vi "电源FGV.vi"(8 "error in (no error)":errorcluster caption="错误输入（无错误）", 9 "Voltage":dbl=2.7, 10 "枚举":T1) -> (0 "error out":errorcluster caption="错误输出", 3 "VISA资源名称输出":refnum<visa-resource-name>)   [LabVIEW 2012]
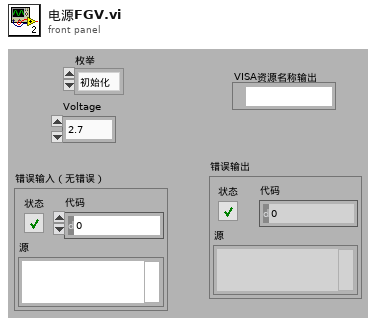
[diagram p1: front panel]
types:
  T1 = typedef "控件 3.ctl" = enum16{"初始化", "读取", "写入", "退出"}
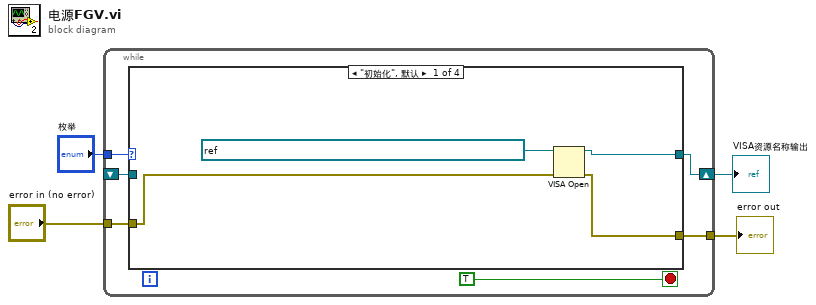
[diagram p0: block diagram]
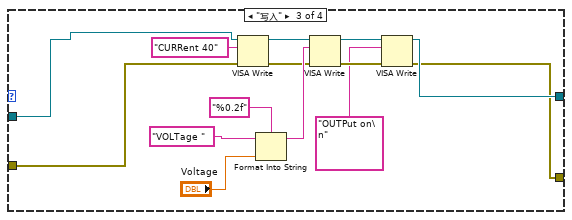
[diagram p3: hidden frame]
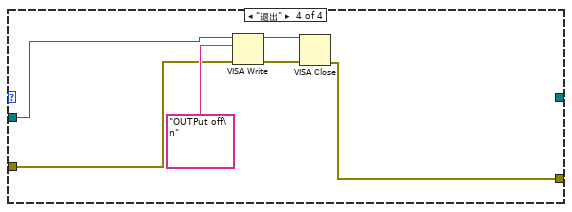
[diagram p4: hidden frame]
diagram:
  n1 = while {
    tunnel: "枚举" -> [w9]
    shift-right: [w8] -> w3
    shift-left: _ -> [w7]
    tunnel: "error in (no error)" -> [w6]
    tunnel: [w5] -> w1
    stop <- TRUE stop-if-true
    n2 = case shown="\"初始化\", 默认" w9 {
      tunnel: [w13 w16 w23 _] -> w8
      tunnel: w7 -> [_ w16 w18 w33]
      tunnel: w6 -> [w12 w15 w17 w32]
      tunnel: [w11 w15 w22 w31] -> w5
      frame "初始化", Default {
        n3 = VISA Open(error in (no error)=w12, VISA resource name=refnum<visa-resource-name> "USB0::0xFFFF::0x6500::600264012697220016::INSTR" ("VISA资源名称")) -> (VISA resource name=w13:refnum<visa-resource-name>, error out=w11:errorcluster)  [unwired: 3 in]
      }
      frame "读取" {
      }
      frame "写入" {
        n4 = VISA Write(VISA resource name=w18, write buffer="CURRent 40" ("写入缓冲区"), error in (no error)=w17) -> (VISA resource name out=w20:refnum<visa-resource-name>, error out=w19:errorcluster)  [unwired: 1 out]
        n5 = Format Into String(format string="%0.2f", initial string="VOLTage " ("format string"), "Voltage") -> (resulting string=w27:string)  [unwired: 1 in, 1 out]
        n6 = VISA Write(VISA resource name=w20, write buffer=w27, error in (no error)=w19) -> (VISA resource name out=w26:refnum<visa-resource-name>, error out=w25:errorcluster)  [unwired: 1 out]
        n7 = VISA Write(VISA resource name=w26, write buffer="OUTPut on\n", error in (no error)=w25) -> (VISA resource name out=w23:refnum<visa-resource-name>, error out=w22:errorcluster)  [unwired: 1 out]
      }
      frame "退出" {
        n8 = VISA Write(VISA resource name=w33, write buffer="OUTPut off\n", error in (no error)=w32) -> (VISA resource name out=w36:refnum<visa-resource-name>, error out=w35:errorcluster)  [unwired: 1 out]
        n9 = VISA Close(VISA resource name=w36, error in (no error)=w35) -> (error out=w31:errorcluster)
      }
    }
  }
  "VISA资源名称输出" <- w3
  "error out" <- w1
